vi "Measure.vi"(8 "error in (no error)":errorcluster, 11 "Measurement in":refnum<class "Measurement.lvclass">) -> (0 "error out":errorcluster, 3 "Measurement out":refnum<class "Measurement.lvclass">)   [LabVIEW 2015, in "Measurement Actor.lvlib" / "Measurement.lvclass"]
uses:
  Measurement.lvclass
  Measurement.lvclass/Measurement.ctl
  <vilib>/ActorFramework/Actor/Actor.lvclass/Actor.ctl
  <vilib>/ActorFramework/Message Enqueuer/Message Enqueuer.lvclass/Message Enqueuer.ctl
  <vilib>/ActorFramework/Message Enqueuer/Init from Existing Queue.vi
  <vilib>/ActorFramework/Message Enqueuer/Enqueue.vi
  <vilib>/ActorFramework/Message Priority Queue/Priority Enqueue.vi
  <vilib>/ActorFramework/Message Enqueuer/Message Enqueuer.lvclass
  Results/Results.lvclass
  Messages/Close Msg/Close Msg.lvclass
  Controller/Messages/Send Results Object/Send Results Object.lvclass
  <vilib>/ActorFramework/Actor/Actor.lvclass
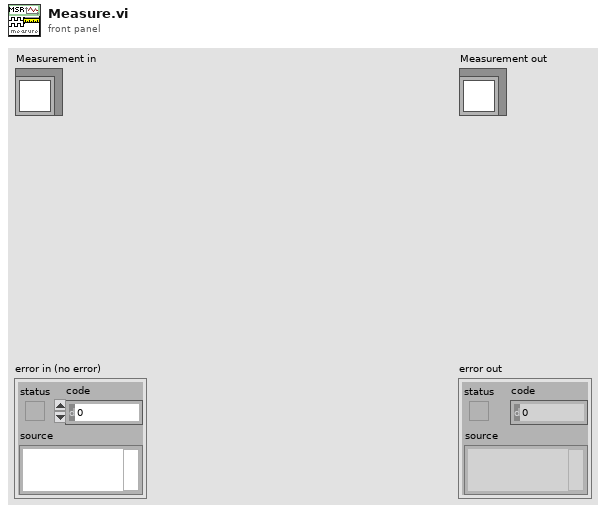
[diagram p1: front panel]
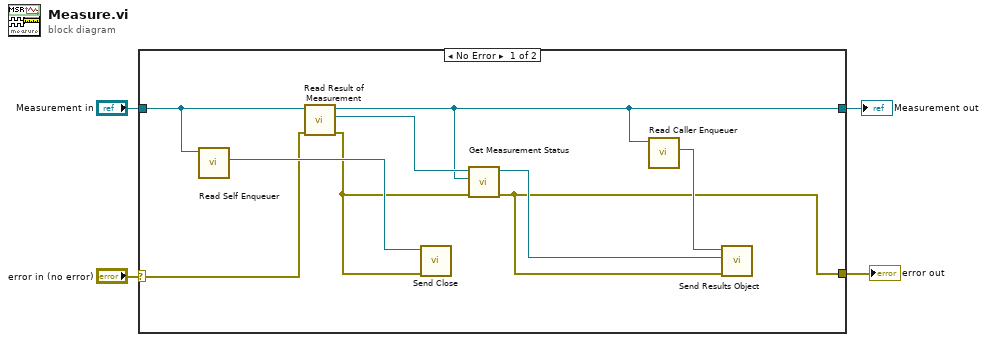
[diagram p0: block diagram]
diagram:
  n1 = case shown="No Error" "error in (no error)" {
    selector: "error in (no error)" -> [w7 w15]
    tunnel: [w5 w15] -> w3
    tunnel: [w8 w14] -> w1
    tunnel: "Measurement in" -> [w10 w14]
    frame No Error {
      n2 = call <vilib>:"Read Self Enqueuer.vi"("Actor"=w10) -> ("Self Enqueuer"=w11:refnum<class "Message Enqueuer.lvclass">)  [unwired: 10 in]
      n3 = call "Read Result of Measurement.vi"("error in (no error)"=w7, "Measurement in"=w10) -> ("error out"=w6:errorcluster, "Result Actor.lvlib:Results.lvclass"=w9:refnum<class "Results.lvclass">, "Measurement out"=w8:refnum<class "Measurement.lvclass">)  [unwired: 7 in]
      n4 = call "Send Close.vi"("error in (no error)"=w6, "Message Enqueuer in"=w11) -> ()  [unwired: 8 in, 2 out]
      n5 = call-dynamic "Get Measurement Status.vi"("error in (no error)"=w6, "Measurement.lvclass"=w8, "Results in"=w9) -> ("error out"=w5:errorcluster, "Results out"=w13:refnum<class "Results.lvclass">)  [unwired: 7 in]
      n6 = call <vilib>:"Read Caller Enqueuer.vi"("Actor"=w8) -> ("Caller Enqueuer"=w12:refnum<class "Message Enqueuer.lvclass">)  [unwired: 10 in]
      n7 = call "Send Results Object.vi"("error in (no error)"=w5, "Results.lvclass"=w13, "Message Enqueuer in"=w12) -> ()  [unwired: 7 in, 2 out]
    }
    frame Error {
    }
  }
  "error out" <- w3
  "Measurement out" <- w1
